vi "Snap And Save.vi"() -> ()   [LabVIEW 8.6]
uses:
  <vilib>/vision/driver/NI_Vision_Acquisition_Software.lvlib
  Program Files/National Instruments/LabVIEW 2009/resource/objmgr/imaqdx.rc
  <vilib>/userdefined/High Color/IMAQdx.ctl
panel:
  out "Image":T1(plugin-control)
  in  "Gain":i64(slide) scale=0.0..24.0
  in  "Exposure Time (ms)":dbl
  in  "Camera Name":T2
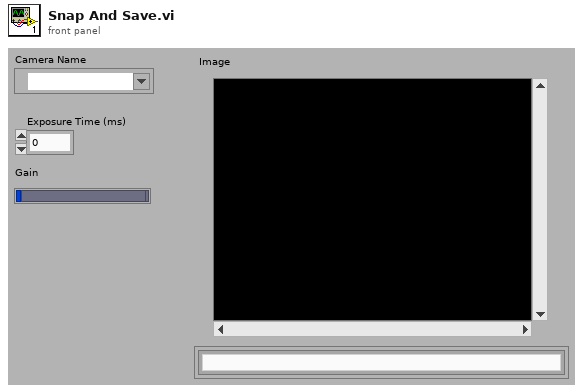
[diagram p1: front panel]
types:
  T1 = typedef "IMAQ Image.ctl" = refnum<image>
  T2 = typedef "IMAQdx.ctl" = refnum<k21>
  T3 = enum32{"Gray", "Binary", "Gradient", "Rainbow", "Temperature"}
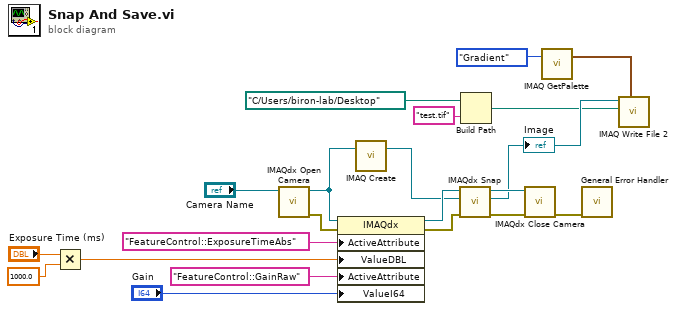
[diagram p0: block diagram]
diagram:
  n1 = Multiply(x="Exposure Time (ms)", y=1000.0) -> (x*y=w15:dbl)
  n2 = call <vilib>:"IMAQdx Open Camera.vi"("Session In"="Camera Name") -> ("error out"=w20:errorcluster, "Session Out"=w12:T2)  [unwired: 2 in, 7 out]
  n3 = property class="IMAQdx"(reference=w12, error in=w20, "ActiveAttribute"="FeatureControl::ExposureTimeAbs", "ValueDBL"=w15, "ActiveAttribute"="FeatureControl::GainRaw", "ValueI64"="Gain") -> (reference out=w11:T2, error out=w13:errorcluster)
  n4 = call "IMAQ Create"("Image Name"=w12) -> ("New Image"=w10:T1)  [unwired: 3 in, 2 out]
  n5 = call <vilib>:"IMAQdx Snap.vi"("error in"=w13, "Image In"=w10, "Session In"=w11) -> ("error out"=w9:errorcluster, "Image Out"=w7:T1, "Session Out"=w8:T2)  [unwired: 6 in]
  "Image" <- w7
  n6 = Build Path(base path=path "C:/Users/biron-lab/Desktop", name or relative path="test.tif") -> (appended path=w1:path)
  n7 = call <vilib>:"IMAQdx Close Camera.vi"("error in"=w9, "Session In"=w8) -> ("error out"=w6:errorcluster)  [unwired: 9 out]
  n8 = call "IMAQ GetPalette"("Palette Number (gray)"=T3."Gradient") -> ("Color Palette"=w5:cluster{"Red":u8, "Green":u8, "Blue":u8}[])  [unwired: 4 in, 1 out]
  n9 = call <vilib>:"General Error Handler.vi"("error in (no error)"=w6) -> ()  [unwired: 1 in, 14 out]
  n10 = call-poly "IMAQ Write File 2"("Color Palette"=w5, "File Path"=w1, "Image"=w7) -> ()  [unwired: 7 in, 2 out]
